vi "Close.vi"(8 "error in (no error)":errorcluster, 11 "Data in":refnum<class "OnChange_Boolean.lvclass">) -> (0 "error out":errorcluster, 3 "Data out":refnum<class "OnChange_Boolean.lvclass">)   [LabVIEW 2021, in "OnChange_Boolean.lvclass"]
doc: "Abstract Data Classes 2.1.1.13\nTim Streeter - TSA\nCopyright (c) 2025, TSA"
uses:
  OnChange_Boolean.lvclass
  OnChange_Boolean.lvclass/OnChange_Boolean.ctl
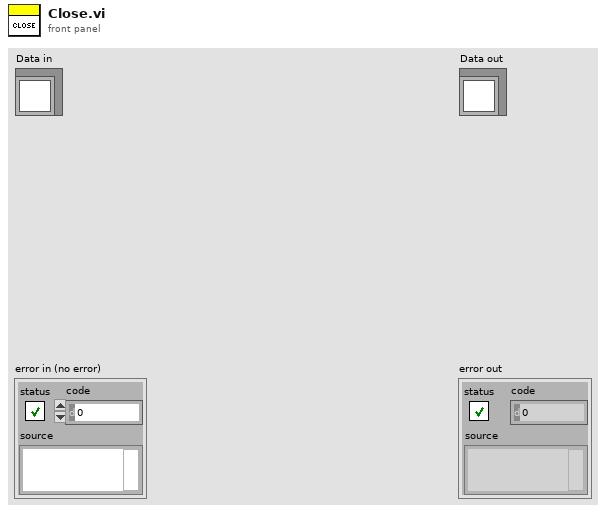
[diagram p1: front panel]
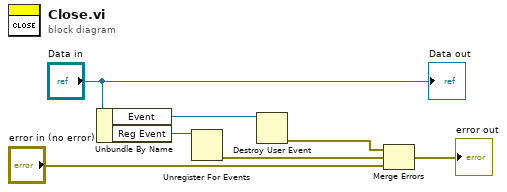
[diagram p0: block diagram]
diagram:
  n1 = Unbundle By Name("Data in") -> ("Event"=w7:refnum<user-event>, "Reg Event"=w5:refnum<event-registration>)
  n2 = Unregister For Events(event registration refnum=w5) -> (error out=w3:errorcluster)  [unwired: 1 in]
  n3 = Destroy User Event(user event=w7) -> (error out=w4:errorcluster)  [unwired: 1 in]
  n4 = Merge Errors(w4, w3, "error in (no error)") -> (→"error out":errorcluster)
  "Data out" <- "Data in"
